vi "download.vi"(8 "error in (no error)":errorcluster, 10 "target_path":path, 11 "address":string) -> (0 "error out":errorcluster, 3 "filepath":path)   [LabVIEW 2015, in "lv-bin-wget.lvlib" / "v1.lvlib"]
uses:
  v1.lvlib
  <userlib>/antonio-alexander/lv-bin/public/api/v1/v1.lvlib
  lv-bin-wget.lvlib
panel:
  in  "quiet?":bool=TRUE
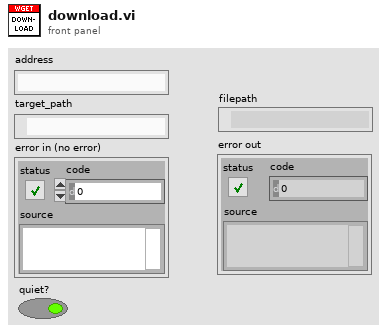
[diagram p1: front panel]
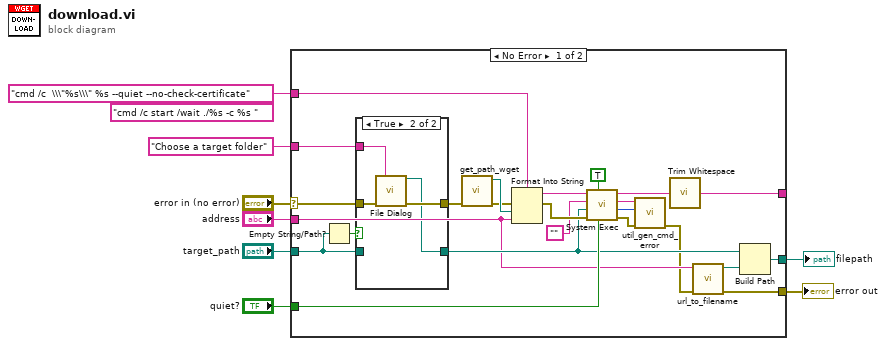
[diagram p0: block diagram]
diagram:
  (unwired) "cmd /c start /wait ./%s -c %s " ("format string")
  n1 = case shown="No Error" "error in (no error)" {
    selector: "error in (no error)" -> [w28 w39]
    tunnel: [w11 w39] -> w7
    tunnel: "target_path" -> [w27 _]
    tunnel: "Choose a target folder" ("prompt") -> [w25 _]
    tunnel: "quiet?" -> [w23 _]
    tunnel: [w19 _] -> _
    tunnel: "address" -> [w13 _]
    tunnel: "cmd /c  \\\"%s\\\" %s --quiet --no-check-certificate" ("format string") -> [w18 _]
    tunnel: [w9 _] -> w1
    frame No Error {
      n2 = Empty String/Path?(string/path=w27) -> (empty?=w26:bool)
      n3 = case shown="True" w26 {
        tunnel: w28 -> [w33 w38]
        tunnel: [w33 w37] -> w16
        tunnel: w27 -> [w34 _]
        tunnel: w25 -> [_ w36]
        tunnel: [w34 w35] -> w14
        frame False {
        }
        frame True {
          n4 = call "File Dialog"("prompt"=w36, "error in"=w38) -> ("selected path"=w35:path, "error out"=w37:errorcluster)  [unwired: 10 in, 2 out]
        }
      }
      n5 = call "get_path_wget.vi"("error in (no error)"=w16) -> ("error out"=w15:errorcluster, "wget"=w17:path)  [unwired: 9 in]
      n6 = Format Into String(format string=w18, error in=w15, w17, w13) -> (resulting string=w31:string, error out=w32:errorcluster)  [unwired: 1 in]
      n7 = call <vilib>:"System Exec.vi"("run minimized? (F)"=w23, "wait until completion? (T)"=TRUE, "error in (no error)"=w32, "working directory"=w14, "standard input"="", "command line"=w31) -> ("error out"=w24:errorcluster, "return code"=w20:i32, "standard error"=w22:string, "standard output"=w21:string)  [unwired: 2 in]
      n8 = call <userlib>:"util_gen_cmd_error.vi"("error in (no error)"=w24, "return_code"=w20, "standard_error"=w22) -> ("error out"=w12:errorcluster)  [unwired: 8 in]
      n9 = call <vilib>:"Trim Whitespace.vi"("string"=w21) -> ("trimmed string"=w19:string)  [unwired: 1 in]
      n10 = call "url_to_filename.vi"("error in (no error)"=w12, "url"=w13) -> ("error out"=w11:errorcluster, "filename"=w10:path)  [unwired: 8 in]
      n11 = Build Path(base path=w14, name or relative path=w10) -> (appended path=w9:path)
    }
    frame Error {
    }
  }
  "error out" <- w7
  "filepath" <- w1
